vi "Close Video Writer.vi"(0 "video writer in":refnum<class "MSC Video Writer.lvclass">, 5 "error in (no error)":errorcluster) -> (14 "video writer out":refnum<class "MSC Video Writer.lvclass">, 19 "error out":errorcluster)   [LabVIEW 2014, in "MSC Video Writer.lvclass"]
uses:
  MSC Video Writer.lvclass
  MSC Video Writer.lvclass/MSC Video Writer.ctl
  Dependencies/x86/MSC I Process32.dll
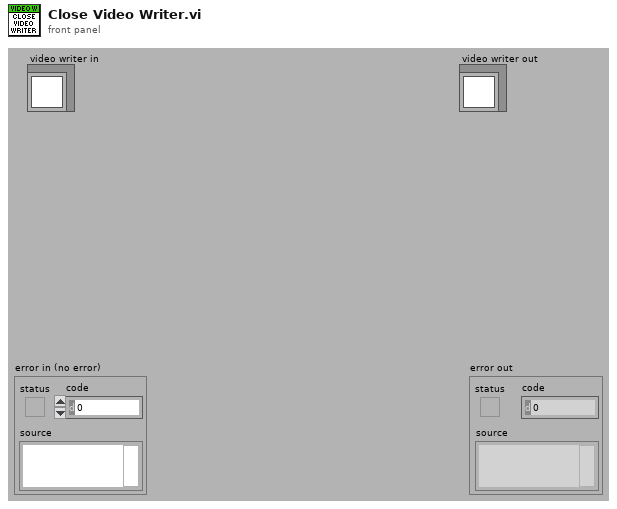
[diagram p1: front panel]
types:
  T1 = typedef "MSC Video Writer.lvclass/Video Writer.ctl" = cluster{"Pointer":u64, "FPS":u32, "Path":path, "FourCC Codec":string, "Size":T2, "Type":T3}
  T2 = typedef "MSC Image.lvclass/Size.ctl" = cluster{"Cols":i32, "Rows":i32}
  T3 = typedef "MSC Image.lvclass/Image Type.ctl" = i32
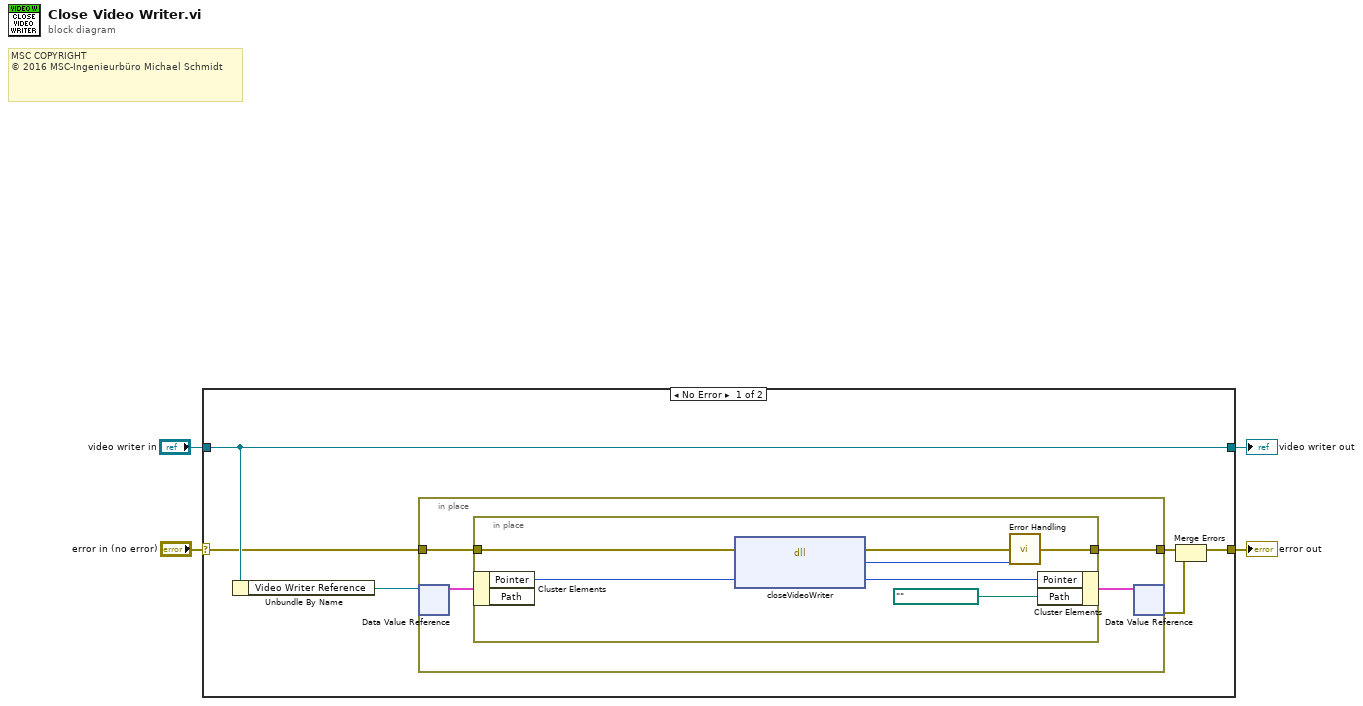
[diagram p0: block diagram]
diagram:
  # "MSC COPYRIGHT\n© 2016 MSC-Ingenieurbüro Michael Schmidt"
  # "MSC COPYRIGHT\n© 2016 MSC-Ingenieurbüro Michael Schmidt"
  n1 = case shown="No Error" "error in (no error)" {
    selector: "error in (no error)" -> [w6 w23]
    tunnel: [w5 w23] -> w3
    tunnel: [w10 w22] -> w1
    tunnel: "video writer in" -> [w10 w22]
    frame No Error {
      n2 = Unbundle By Name(w10) -> ("Video Writer Reference"=w7:refnum<data-value>)
      n3 = in-place {
        in-place-border: [w12] -> w8
        in-place-border: w6 -> [w11]
        n4 = in-place-dvr #1(w7) -> (w13:T1)  [unwired: 1 out]
        n5 = in-place {
          in-place-border: [w18] -> w12
          in-place-border: w11 -> [w21]
          n6 = in-place-cluster #2(w13) -> ("Pointer"=w17:u64)  [unwired: 1 out]
          n7 = dll-call lib="C:/Users/MSC/LabVIEW Projekte/LV 2014/MSC I-Process/user.lib/MSC-I Process/Dependencies/x86/MSC I Process*.dll" fn="closeVideoWriter"(error in=w21, "writerPointer"=w17) -> (error out=w19:errorcluster, "error"=w20:i32, "writerPointer"=w16:u64)  [unwired: 2 in, 1 out]
          n8 = call "Error Handling.vi"("error in (no error)"=w19, "return type"=w20) -> ("error out"=w18:errorcluster)  [unwired: 12 in, 1 out]
          n9 = in-place-cluster #2("Pointer"=w16, "Path"=path "") -> (w14:T1)
        }
        n10 = in-place-dvr #1(w14) -> (w9:errorcluster)  [unwired: 1 out]
      }
      n11 = Merge Errors(w8, w9) -> (w5:errorcluster)
    }
    frame Error {
    }
  }
  "error out" <- w3
  "video writer out" <- w1
